vi "Read Plot Area Bounds.vi"(9 "GraphChart in":refnum<class "GraphChart.lvclass">) -> (3 "GraphChart out":refnum<class "GraphChart.lvclass">, 4 "Plot Area Bounds":T1)   [LabVIEW 2014, in "Raspberry Pi Compatible Compiler for LabVIEW.lvlib" / "GraphChart.lvclass"]
uses:
  GraphChart.lvclass
  GraphChart.lvclass/GraphChart.ctl
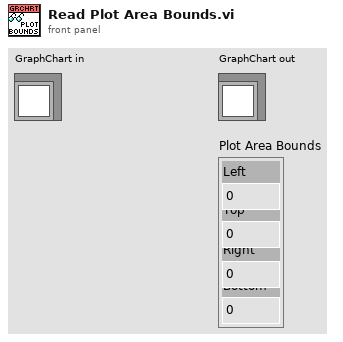
[diagram p1: front panel]
types:
  T1 = cluster{"Left":i16, "Top":i16, "Right":i16, "Bottom":i16}
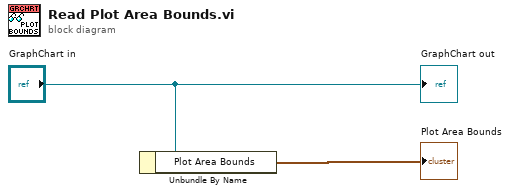
[diagram p0: block diagram]
diagram:
  n1 = Unbundle By Name("GraphChart in") -> ("Plot Area Bounds"=→"Plot Area Bounds":T1)
  "GraphChart out" <- "GraphChart in"
